vi "find_builders.vi"(8 "error in (no error)":errorcluster, 11 "folder":path) -> (0 "error out":errorcluster, 1 "name []":string[](array[string]), 2 "lv-builder []":refnum<class "lv-builder.lvclass">[](array[class]), 3 "path []":path[](array[path]))   [LabVIEW 2015, in "lv-builder.lvlib"]
uses:
  lv-builder.lvlib
  lv-builder.lvclass
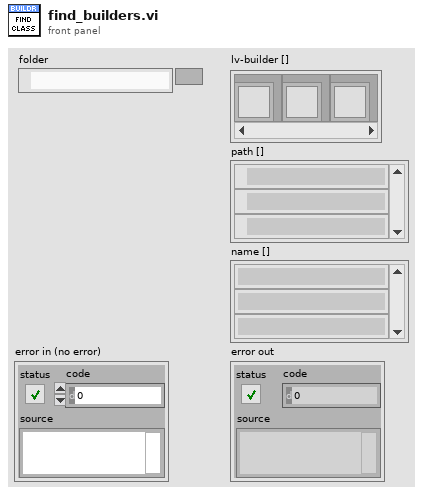
[diagram p1: front panel]
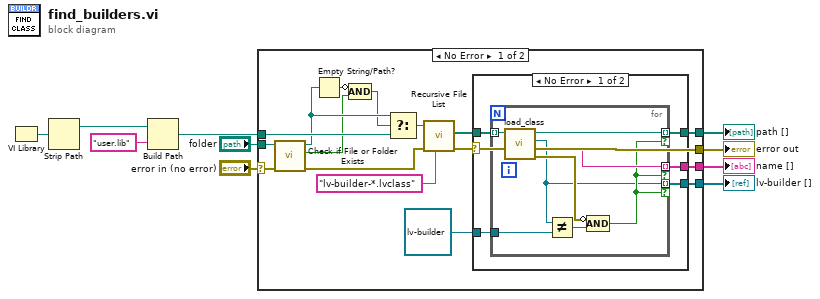
[diagram p0: block diagram]
diagram:
  n1 = VI Library() -> (path=w5:path)
  n2 = Strip Path(path=w5) -> (stripped path=w3:path)  [unwired: 1 out]
  n3 = Build Path(base path=w3, name or relative path="user.lib") -> (appended path=w2:path)
  n4 = case shown="No Error" "error in (no error)" {
    selector: "error in (no error)" -> [w20 w40]
    tunnel: [w24 _] -> w9
    tunnel: [w23 w40] -> w8
    tunnel: "folder" -> [w19 _]
    tunnel: [w22 _] -> w6
    tunnel: w2 -> [w17 _]
    tunnel: [w21 _] -> w1
    frame No Error {
      n5 = call <vilib>:"Check if File or Folder Exists.vi"("error in (no error)"=w20, "path"=w19) -> ("error out"=w18:errorcluster, "file or folder exists?"=w12:bool, "dup path"=w15:path)  [unwired: 7 in]
      n6 = Empty String/Path?(string/path=w15) -> (empty?=w14:bool)
      n7 = Compound Arithmetic op=AND(invert w14, w12) -> (w13:bool)
      n8 = Select(t=w15, s=w13, f=w17) -> (s? t:f=w16:path)
      n9 = call <vilib>:"Recursive File List.vi"("pattern"="lv-builder-*.lvclass", "error in (no error)"=w18, "Folder Path"=w16) -> ("error out"=w23:errorcluster, "All Files in Dir"=w25:path[])  [unwired: 4 in, 3 out]
      n10 = case shown="No Error" w23 {
        tunnel: w25 -> [w31 _]
        tunnel: [w30 _] -> w24
        tunnel: [w29 _] -> w22
        tunnel: [w28 _] -> w21
        tunnel: refnum<class "lv-builder.lvclass"> refnum ("lv-build.lvlib:lv-build.lvclass") -> [w27 _]
        frame No Error {
          n11 = for {
            tunnel: w31 -> [w37] mode=indexing
            tunnel: [w32] -> w30 mode=indexing if=w35
            tunnel: [w36] -> w29 mode=indexing if=w35
            tunnel: [w38] -> w28 mode=indexing if=w35
            tunnel: w27 -> [w33]
            n12 = call "load_class.vi"("builder_class in"=w37) -> ("error out"=w39:errorcluster, "name"=w38:string, "lv_builder"=w32:refnum<class "lv-builder.lvclass">, "builder_class out"=w36:path)  [unwired: 7 in]
            n13 = Not Equal?(x=w32, y=w33) -> (x != y?=w34:bool)
            n14 = Compound Arithmetic op=AND(invert w39, w34) -> (w35:bool)
          }
        }
        frame Error {
        }
      }
    }
    frame Error {
    }
  }
  "error out" <- w8
  "lv-builder []" <- w9
  "path []" <- w6
  "name []" <- w1
